vi "Fetch Measurement (Time Interval Error).vi"(0 "VISA resource name":refnum<visa-resource-name>, 1 "Direction (0: Rising)":i32(ring) items=["Rising", "Falling", "Both"], 2 "Units (0: Second)":i32(ring) items=["Second", "Unit Interval"], 5 "Channel (1: Channel 1)":i32(ring)=1 items=["Channel 1"=1, "Channel 2"=2, "Channel 3"=3, "Channel 4"=4, "Function 1"=5, "Function 2"=6, "Function 3"=7, "Function 4"=8, "Memory 1"=9, "Memory 2"=10, "Memory 3"=11, "Memory 4"=12], 7 "Measurement Function (0: Time Interval Error (Data))":i32(ring) items=["Time Interval Error (Data)", "Time Interval Error (Clock)"], 11 "error in (no error)":errorcluster) -> (4 "VISA resource name out":refnum<visa-resource-name>, 6 "Time Interval Error (s)":dbl, 15 "error out":errorcluster)   [LabVIEW 2012, in "Agilent 8000 Series.lvlib"]
doc: "Obtains a waveform measurement (Time Interval Error) and returns the measurement value. The waveform on which the oscilloscope calculates the waveform measurement is from an acquisition that you previously initiated. \n\nUse the Initiate Acquisition.vi to start an acquisition on the channels that you enable with the Configure Channel.vi. The oscilloscope acquires waveforms for the enabled channels concurrently. You use the Wait For Operation Complete.vi to wait for operation complete. You call this VI separately for each waveform measurement you want to obtain on a specific channel.\n\nYou can call the Read Measurement.vi instead of the Initiate Acquisition.vi. The Read Measurement.vi starts an acquisition on all enabled channels. It then waits for the acquisition to complete, obtains a waveform measurement on the channel you specify, and returns the measurement value. You call this VI separately for any other waveform measurement that you want to obtain on a specific channel.\n\nNotes:\n\n(1) You must configure the appropriate reference levels before you call this VI to take measurement.\n\n(2) You configure the low, mid, and high references either by calling the Configure Reference Levels.vi.\n\n(3) This VI does not check the instrument status. Typically, you call this VI only in a sequence of calls to other low-level driver VIs. The sequence performs one operation. You use the low-level VIs to optimize one or more aspects of interaction with the instrument. If you want to check the instrument status, call the Error-Query.vi at the conclusion of the sequence."
uses:
  <instrlib>/Agilent 8000 Series/Agilent 8000 Series.lvlib
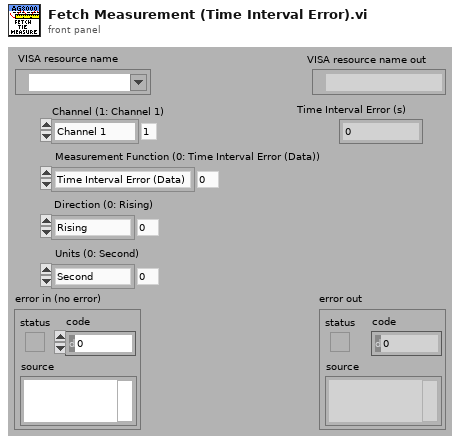
[diagram p1: front panel]
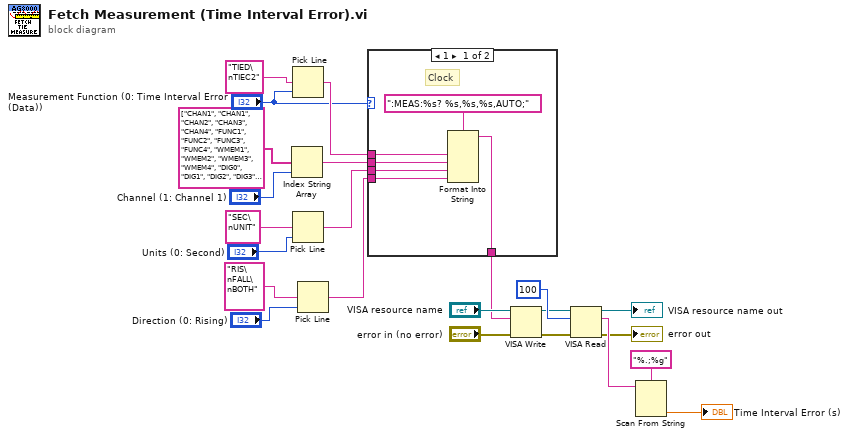
[diagram p0: block diagram]
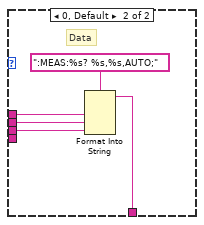
[diagram p2: hidden frame]
diagram:
  n1 = Index String Array(1:"Channel (1: Channel 1)", 2:string[] ["CHAN1", "CHAN1", "CHAN2", "CHAN3", "CHAN4", "FUNC1", "FUNC2", "FUNC3", "FUNC4", "WMEM1", "WMEM2", "WMEM3", "WMEM4", "DIG0", "DIG1", "DIG2", "DIG3", "DIG4", "DIG5", "DIG6", "DIG7", "DIG8", "DIG9", "DIG10", "DIG11", "DIG12", "DIG13", "DIG14", "DIG15", "AUX", "LINE"]) -> (0:w20:string)  [unwired: 1 in]
  n2 = Pick Line(multi-line string="TIED\nTIEC2", line index="Measurement Function (0: Time Interval Error (Data))") -> (output string=w18:string)  [unwired: 1 in]
  n3 = Pick Line(multi-line string="SEC\nUNIT", line index="Units (0: Second)") -> (output string=w23:string)  [unwired: 1 in]
  n4 = Pick Line(multi-line string="RIS\nFALL\nBOTH", line index="Direction (0: Rising)") -> (output string=w12:string)  [unwired: 1 in]
  n5 = case shown="1" "Measurement Function (0: Time Interval Error (Data))" {
    tunnel: w18 -> [w28 w33]
    tunnel: w20 -> [w27 w32]
    tunnel: [w26 w31] -> w4
    tunnel: w23 -> [w25 w30]
    tunnel: w12 -> [w24 _]
    frame 1 {
      # "Clock"
      n6 = Format Into String(format string=":MEAS:%s? %s,%s,%s,AUTO;", w28, w27, w25, w24) -> (resulting string=w26:string)  [unwired: 2 in, 1 out]
    }
    frame 0, Default {
      # "Data"
      n7 = Format Into String(format string=":MEAS:%s? %s,%s,AUTO;", w33, w32, w30) -> (resulting string=w31:string)  [unwired: 2 in, 1 out]
    }
  }
  n8 = VISA Write(VISA resource name="VISA resource name", write buffer=w4, error in (no error)="error in (no error)") -> (VISA resource name out=w7:refnum<visa-resource-name>, error out=w8:errorcluster)  [unwired: 1 out]
  n9 = VISA Read(VISA resource name=w7, byte count=u32 100, error in (no error)=w8) -> (VISA resource name out=→"VISA resource name out":refnum<visa-resource-name>, read buffer=w10:string, error out=→"error out":errorcluster)  [unwired: 1 out]
  n10 = Scan From String(format string="%.;%g", input string=w10) -> (output 1=→"Time Interval Error (s)":dbl)  [unwired: 3 in, 3 out]
